vi "Generator bazat pe modulul Sine Waveform.vi"() -> ()   [LabVIEW 2011]
uses:
  <vilib>/measure/NI_MABase.lvlib
panel:
  in  "phase":dbl
  in  "amplitude":dbl
  in  "frequency":dbl
  in  "offset":dbl
  in  "Sampling 0":cluster{"Fs":dbl, "#s":dbl}
  in  "error in":errorcluster
  out "error out":errorcluster
  out "Waveform Graph":waveform(dbl)(graph)
  in  "reset signal":bool
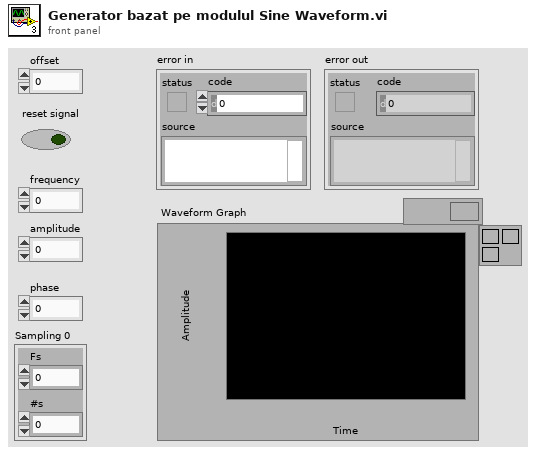
[diagram p1: front panel]
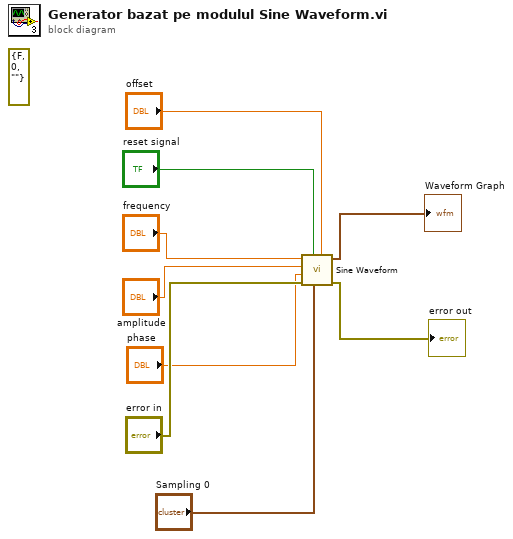
[diagram p0: block diagram]
diagram:
  (unwired) errorcluster {"status"=FALSE, "code"=0, "source"=""} ("error out")
  n1 = call <vilib>:"Sine Waveform.vi"("offset"="offset", "sampling info"="Sampling 0", "reset signal"="reset signal", "error in (no error)"="error in", "phase"="phase", "amplitude"="amplitude", "frequency"="frequency") -> ("error out"=→"error out":errorcluster, "signal out"=→"Waveform Graph":waveform(dbl))  [unwired: 3 in]
